vi "offsets.vi"() -> ()   [LabVIEW 2013]
panel:
  out "offsets":cluster{"xr":dbl, "xl":dbl, "yu":dbl, "yd":dbl}
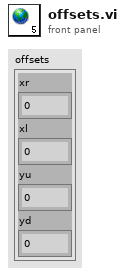
[diagram p1: front panel]
diagram:
